vi "subvi2.vi"() -> (3 "VI Path":path)   [LabVIEW 2017]
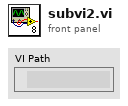
[diagram p1: front panel]
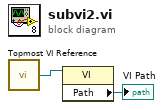
[diagram p0: block diagram]
diagram:
  n1 = call "Topmost VI Reference.vi"() -> ("Topmost VI's Reference"=w2:refnum<vi>)  [unwired: 5 in]
  n2 = property class="VI"(reference=w2) -> ("Path"=→"VI Path":path)  [unwired: 1 in, 2 out]
